vi "Set Slot.vi"(8 "error in":errorcluster, 10 "module":refnum<class "Module.lvclass">, 11 "slot ref in":T2 format="%.0x") -> (0 "error out":errorcluster, 3 "slot ref out":T2 format="%.0x")   [LabVIEW 2017, in "Scan Engine Scripting.lvlib"]
uses:
  Scan Engine Scripting.lvlib
  Modules.lvlibp/niveristand-scan-engine-module-libraries/Source/RSI Module/RSI Module.lvclass
  Modules.lvlibp
  <vilib>/NI Veristand/Custom Device API/Custom Device API.lvlib
  Scan Engine Custom Device.lvlib
  Modules/Module/Module.lvclass
  Modules.lvlibp/niveristand-scan-engine-ethercat-custom-device/Custom Device Source/Scripting/Modules/Module/Module.lvclass
  <vilib>/NI Veristand/Custom Device API/Custom Device Item Ref.ctl
  Modules.lvlibp/niveristand-scan-engine-module-libraries/Source/RSI Module/Module Models.ctl
panel:
  in  "module model":T1
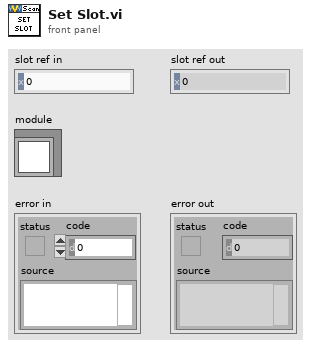
[diagram p1: front panel]
types:
  T1 = typedef "Modules.lvlibp/RSI Module.lvclass/Module Models.ctl" = enum16{"Empty", "NI 9201", "NI 9203", "NI 9205", "NI 9206", "NI 9207", "NI 9208", "NI 9209", "NI 9210", "NI 9211", "NI 9212", "NI 9213", "NI 9214", "NI 9215", "NI 9216", "NI 9217", "NI 9219", "NI 9220", "NI 9221", "NI 9222", "NI 9223", "NI 9224", "NI 9225", "NI 9226", "NI 9227", "NI 9228", "NI 9229", "NI 9233", "NI 9234", "NI 9235", "NI 9236", "NI 9237", "NI 9239", "NI 9242", "NI 9244", "NI 9253", "NI 9263", "NI 9264", "NI 9265", "NI 9266", "NI 9269", "NI 9344", "NI 9350", "NI 9375", "NI 9401", "NI 9402", "NI 9403", "NI 9411", "NI 9421", "NI 9422", "NI 9423", "NI 9425", "NI 9426", "NI 9435", "NI 9436", "NI 9437", "NI 9472", "NI 9474", "NI 9475", "NI 9476", "NI 9477", "NI 9478", "NI 9481", "NI 9482", "NI 9485"}
  T2 = typedef "Custom Device API.lvlib/Custom Device Item Ref.ctl" = u64
  T3 = typedef "Modules.lvlibp/Custom Device API.lvlib/Custom Device Item Ref.ctl" = u64
  T4 = typedef "Modules.lvlibp/RSI Module.lvclass/Slot Settings.ctl" = cluster{"Slot":u32, "EtherCAT?":bool}
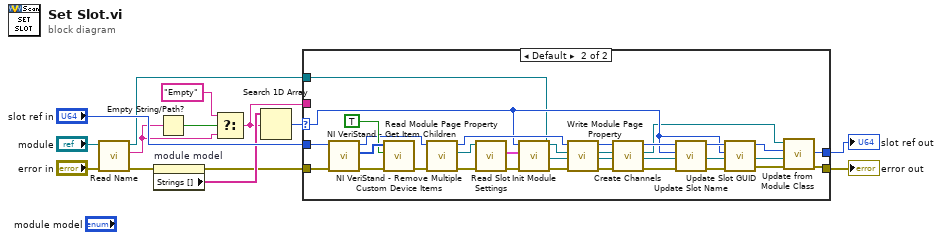
[diagram p0: block diagram]
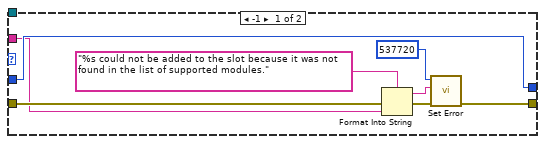
[diagram p2: hidden frame]
diagram:
  n1 = call-dynamic "Read Name.vi"("error in"="error in", "module in"="module") -> ("error out"=w1:errorcluster, "name"=w3:string, "module out"=w2:refnum<class "Module.lvclass">)  [unwired: 7 in]
  n2 = property on="module model" class="Enum (strict)"(error in=w1) -> (error out=w9:errorcluster, "Strings []"=w11:string[])  [unwired: 1 in, 1 out]
  n3 = Empty String/Path?(string/path=w3) -> (empty?=w6:bool)
  n4 = Select(t="Empty" ("f"), s=w6, f=w3) -> (s? t:f=w5:string)
  n5 = Search 1D Array(1D array=w11, element=w5) -> (index of element=w10:i32)  [unwired: 1 in]
  n6 = case shown="Default" w10 {
    selector: w10 -> [_ w29]
    tunnel: "slot ref in" -> [w22 w35]
    tunnel: w9 -> [w19 w34]
    tunnel: [w21 w25] -> w13
    tunnel: [w22 w24] -> w12
    tunnel: w5 -> [w16 _]
    tunnel: w2 -> [_ w23]
    frame -1 {
      n7 = Format Into String(format string="%s could not be added to the slot because it was not found in the list of supported modules.", error in=w19, w16) -> (resulting string=w15:string, error out=w17:errorcluster)  [unwired: 1 in]
      n8 = call "Set Error.vi"("error in (no error)"=w17, "Message"=w15, "Code"=537720) -> ("error out"=w21:errorcluster)  [unwired: 8 in]
    }
    frame Default {
      n9 = call <vilib>:"NI VeriStand - Get Item Children.vi"("error in (no error)"=w34, "Item Ref in"=w35) -> ("error out"=w41:errorcluster, "Child Refs"=w43:T2[], "Item Ref out"=w40:T2)  [unwired: 6 in, 1 out]
      n10 = call <vilib>:"NI VeriStand - Remove Multiple Custom Device Items.vi"("error in (no error)"=w41, "Force Delete (F)"=TRUE, "Item Refs in"=w43) -> ("error out"=w39:errorcluster)  [unwired: 7 in, 1 out]
      n11 = call "Read Module Page Property.vi"("error in (no error)"=w39, "Node Ptr In"=w40) -> ("error out"=w50:errorcluster, "RSI Module"=w49:refnum<class "RSI Module.lvclass">, "Node Ptr Out"=w48:T3)  [unwired: 7 in]
      n12 = call "Read Slot Settings.vi"("error in (no error)"=w50, "RSI Module in"=w49) -> ("error out"=w47:errorcluster, "Slot Settings"=w46:T4)  [unwired: 7 in, 1 out]
      n13 = call "Init Module.vi"("error in (no error)"=w47, "Slot Settings"=w46, "Module Model"=w29) -> ("error out"=w44:errorcluster, "RSI Module out"=w45:refnum<class "RSI Module.lvclass">)  [unwired: 7 in]
      n14 = call "Write Module Page Property.vi"("error in (no error)"=w44, "RSI Module"=w45, "Node Ptr In"=w48) -> ("error out"=w38:errorcluster, "RSI Module out"=w37:refnum<class "RSI Module.lvclass">, "Node Ptr Out"=w36:T3)  [unwired: 6 in]
      n15 = call-dynamic "Create Channels.vi"("error in (no error)"=w38, "RSI Module in"=w37, "Parent Ref in"=w36) -> ("error out"=w33:errorcluster, "RSI Module out"=w28:refnum<class "RSI Module.lvclass">, "Parent Ref out"=w32:T3)  [unwired: 6 in]
      n16 = call "Update Slot Name.vi"("error in"=w33, "module"=w29, "slot ref in"=w32) -> ("error out"=w31:errorcluster, "slot ref out"=w30:T2)  [unwired: 6 in, 1 out]
      n17 = call "Update Slot GUID.vi"("error in"=w31, "module model"=w29, "slot ref in"=w30) -> ("error out"=w26:errorcluster, "slot ref out"=w27:T2)  [unwired: 7 in]
      n18 = call-dynamic "Update from Module Class.vi"("error in"=w26, "module in"=w23, "slot ref in"=w27, "RSI Module in"=w28) -> ("error out"=w25:errorcluster, "slot ref out"=w24:T3)  [unwired: 4 in, 2 out]
    }
  }
  "error out" <- w13
  "slot ref out" <- w12
